vi "Testing DIO Read.vi"() -> ()   [LabVIEW 2020]
uses:
  TypeDefs/TypeDef - Cluster Representing Decoded JSON Message.ctl
panel:
  out "Boolean array":bool[](array[boolean])
  out "Data out":T1
  in  "DAQ IP Address":string="192.168.1.1"
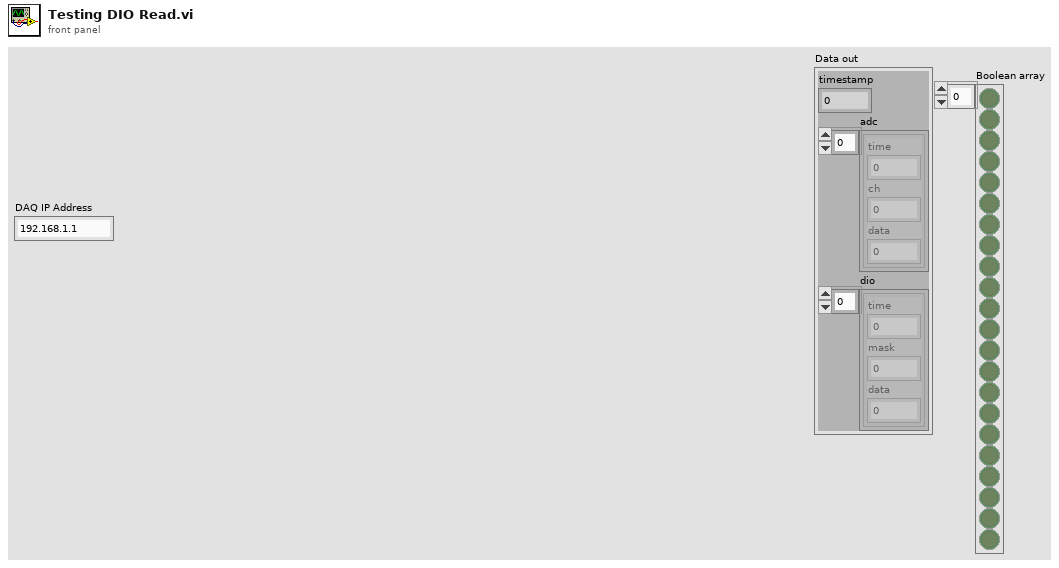
[diagram p1: front panel]
types:
  T1 = typedef "TypeDef - Cluster Representing Decoded JSON Message.ctl" = cluster{"timestamp":u64, "adc":cluster{"time":i32, "ch":i32, "data":i32}[], "dio":cluster{"time":i32, "mask":i32, "data":u16}[]}
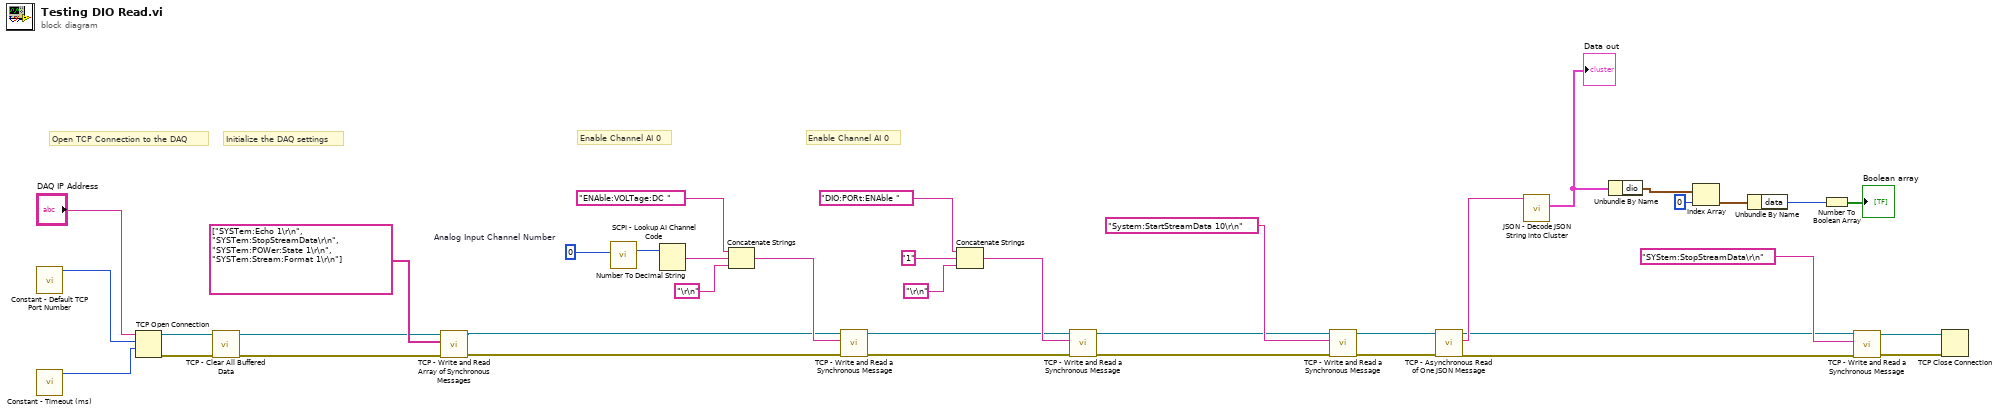
[diagram p0: block diagram]
diagram:
  w27 = 0  # Analog Input Channel Number
  # "Enable Channel AI 0"
  # "Enable Channel AI 0"
  # "Open TCP Connection to the DAQ"
  # "Initialize the DAQ settings"
  n1 = call "Constant - Default TCP Port Number.vi"() -> ("Port"=w38:u16)  [unwired: 11 in]
  n2 = call "Constant - Timeout (ms).vi"() -> ("timeout (ms)"=w33:i32)  [unwired: 11 in]
  n3 = TCP Open Connection(address="DAQ IP Address", remote port or service name=w38, timeout ms (60000)=w33) -> (connection ID=w17:refnum<k5>, error out=w16:errorcluster)  [unwired: 2 in]
  n4 = call "TCP - Clear All Buffered Data.vi"("error in"=w16, "TCP Network Connection in"=w17) -> ("error out"=w15:errorcluster, "TCP Network Connection out"=w14:refnum<k5>)  [unwired: 7 in, 1 out]
  n5 = call "TCP - Write and Read Array of Synchronous Messages.vi"("error in"=w15, "Array of Messages to Send"=string[] ["SYSTem:Echo 1\r\n", "SYSTem:StopStreamData\r\n", "SYSTem:POWer:State 1\r\n", "SYSTem:Stream:Format 1\r\n"], "TCP Network Connection in"=w14) -> ("error out"=w20:errorcluster, "TCP Network Connection out"=w21:refnum<k5>)  [unwired: 6 in, 1 out]
  n6 = call "SCPI - Lookup AI Channel Code.vi"("Analog Input Channel Number"=w27) -> ("Channel Code"=w26:i32)  [unwired: 10 in]
  n7 = Number To Decimal String(number=w26) -> (decimal integer string=w24:string)  [unwired: 1 in]
  n8 = Concatenate Strings("ENAble:VOLTage:DC " ("Message to Send"), w24, "\r\n" ("string")) -> (w22:string)
  n9 = call "TCP - Write and Read a Synchronous Message.vi"("error in"=w20, "Message to Send"=w22, "TCP Network Connection in"=w21) -> ("error out"=w19:errorcluster, "TCP Network Connection out"=w18:refnum<k5>)  [unwired: 6 in, 1 out]
  n10 = Concatenate Strings("DIO:PORt:ENAble " ("Message to Send"), "1" ("string"), "\r\n" ("string")) -> (w34:string)
  n11 = call "TCP - Write and Read a Synchronous Message.vi"("error in"=w19, "Message to Send"=w34, "TCP Network Connection in"=w18) -> ("error out"=w7:errorcluster, "TCP Network Connection out"=w8:refnum<k5>)  [unwired: 6 in, 1 out]
  n12 = call "TCP - Write and Read a Synchronous Message.vi"("error in"=w7, "Message to Send"="System:StartStreamData 10\r\n" ("data in"), "TCP Network Connection in"=w8) -> ("error out"=w29:errorcluster, "TCP Network Connection out"=w30:refnum<k5>)  [unwired: 6 in, 1 out]
  n13 = call "TCP - Asynchronous Read of One JSON Message.vi"("error in"=w29, "TCP Network Connection in"=w30) -> ("error out"=w9:errorcluster, "Received JSON Message"=w28:string, "TCP Network Connection out"=w12:refnum<k5>)  [unwired: 7 in]
  n14 = call "JSON - Decode JSON String into Cluster.vi"("JSON String"=w28) -> ("Data out"=w6:T1)  [unwired: 9 in, 1 out]
  "Data out" <- w6
  n15 = Unbundle By Name(w6) -> ("dio"=w5:cluster{"time":i32, "mask":i32, "data":u16}[])
  n16 = Index Array(array=w5, index=0) -> (element=w3:cluster{"time":i32, "mask":i32, "data":u16})
  n17 = Unbundle By Name(w3) -> ("data"=w2:u16)
  n18 = Number To Boolean Array(number=w2) -> (Boolean array=→"Boolean array":bool[])
  n19 = call "TCP - Write and Read a Synchronous Message.vi"("error in"=w9, "Message to Send"="SYStem:StopStreamData\r\n", "TCP Network Connection in"=w12) -> ("error out"=w10:errorcluster, "TCP Network Connection out"=w11:refnum<k5>)  [unwired: 6 in, 1 out]
  n20 = TCP Close Connection(connection ID=w11, error in (no error)=w10) -> ()  [unwired: 1 in, 2 out]
